vi "Main.vi"(11 "Module Admin":refnum<class "Delacor_lib_QMH_Module Admin.lvclass">) -> ()   [LabVIEW 2021, in "INSTR.lvlib"]
doc: "This template is based off of the Queued Message Handler design pattern and the Queued Message Handler project template that ships with LabVIEW.\n\nThe main difference is that the queue is private to this module and communication between modules is performed via Broadcast and Request events.\n\nRequest events are wrapped in public API methods and are handled in the Event Handling Loop (EHL) of this VI. Any module can register for Broadcast events sent by this module. The EHL generates messages based on user interface actions.\n\nThe Message Handling Loop (MHL) processes messages generated by the EHL, or by other messages. The messages are string values, so new messages can be added easily to the Message Cases case structure in the MHL. Each message cluster can also provide an optional value for Message Data, which is a variant that can be converted to whatever message-specific data is required.\n_____\nBased on Delacor QMH Project Template 5.0.0.82.\n\n<b>Note:</b> This VI was modified by the <b>Validate DQMH Module</b> tool to add a 'Panel Hidden' status updated broadcast to the Panel Close? event when External Launch = TRUE.\n\n<b>Note:</b> This VI was modified by the <b>Validate DQMH Module</b> tool to add a call to the Error Reported VI at the end of the 'Exit' MHL frame."
uses:
  INSTR.lvlib
  <vilib>/Delacor/Delacor QMH/Libraries/Module Admin_class/Delacor_lib_QMH_Module Admin.lvclass
  Module Data--cluster.ctl
  <vilib>/Delacor/Delacor QMH/Libraries/Message Queue_class/Delacor_lib_QMH_Message Queue.lvclass/Delacor_lib_QMH_Message Queue.ctl
  Stop Argument--cluster.ctl
  <vilib>/Delacor/Delacor QMH/Libraries/Module Admin_class/Delacor_lib_QMH_Module Admin.lvclass/Delacor_lib_QMH_Module Admin.ctl
  Simulation Argument--cluster.ctl
  <vilib>/Utility/miscctls.llb/LVPointTypeDef.ctl
  <vilib>/Delacor/Delacor QMH/Libraries/Message Queue_class/Delacor_lib_QMH_Enqueue Message (Single).vi
  <vilib>/Delacor/Delacor QMH/Libraries/Module Admin_class/Delacor_lib_QMH_Get External Launch.vi
  <vilib>/Utility/error.llb/Error Cluster From Error Code.vi
  <vilib>/ErrorRing/Error Ring.xnode
  <vilib>/Delacor/Delacor QMH/Libraries/Message Queue_class/Delacor_lib_QMH_Message Queue.lvclass
  <vilib>/DQMH Consortium/Lumos API/Libraries/SDV API/SDV API.lvlib
panel:
  out "ModuleName":string
  out "Sim?":bool
  in  "ExitMod":bool
  in  "Simulate MHL Error":bool
  in  "Simulate EHL Error":bool
  out "error out":errorcluster
  out "Status":string
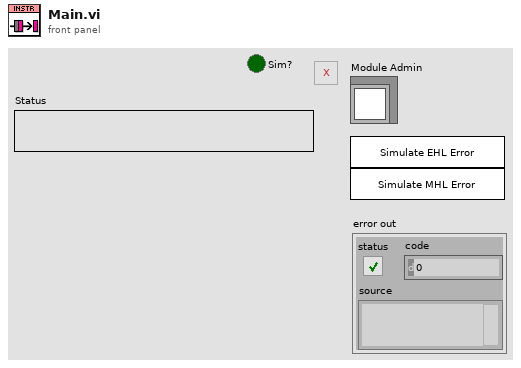
[diagram p1: front panel]
types:
  T1 = typedef "INSTR.lvlib/Request Events--cluster.ctl" = cluster{"Stop Module":refnum<user-event>, "Show Panel":refnum<user-event>, "Hide Panel":refnum<user-event>, "Get Module Execution Status":refnum<user-event>, "Show Diagram":refnum<user-event>, "Simulation":refnum<user-event>}
  T2 = typedef "INSTR.lvlib/Module Data--cluster.ctl" = cluster{"Status":string, "Sim":bool}
  T3 = enum32{"invalid lock state", "Not Locked", "Locked (No Password)", "Password-protected"}
  T4 = typedef "INSTR.lvlib/Stop Argument--cluster.ctl" = cluster{"Origin":string, "Exit via Stop Module Req?":bool, "Wait for Module to stop?":bool}
  T5 = typedef "INSTR.lvlib/Simulation Argument--cluster.ctl" = cluster{"Sim?":bool}
  T6 = typedef "LVPointTypeDef.ctl" = cluster{"Horizontal":i16, "Vertical":i16}
  T7 = enum32{"Invalid", "Standard", "Closed", "Hidden", "Minimized", "Maximized"}
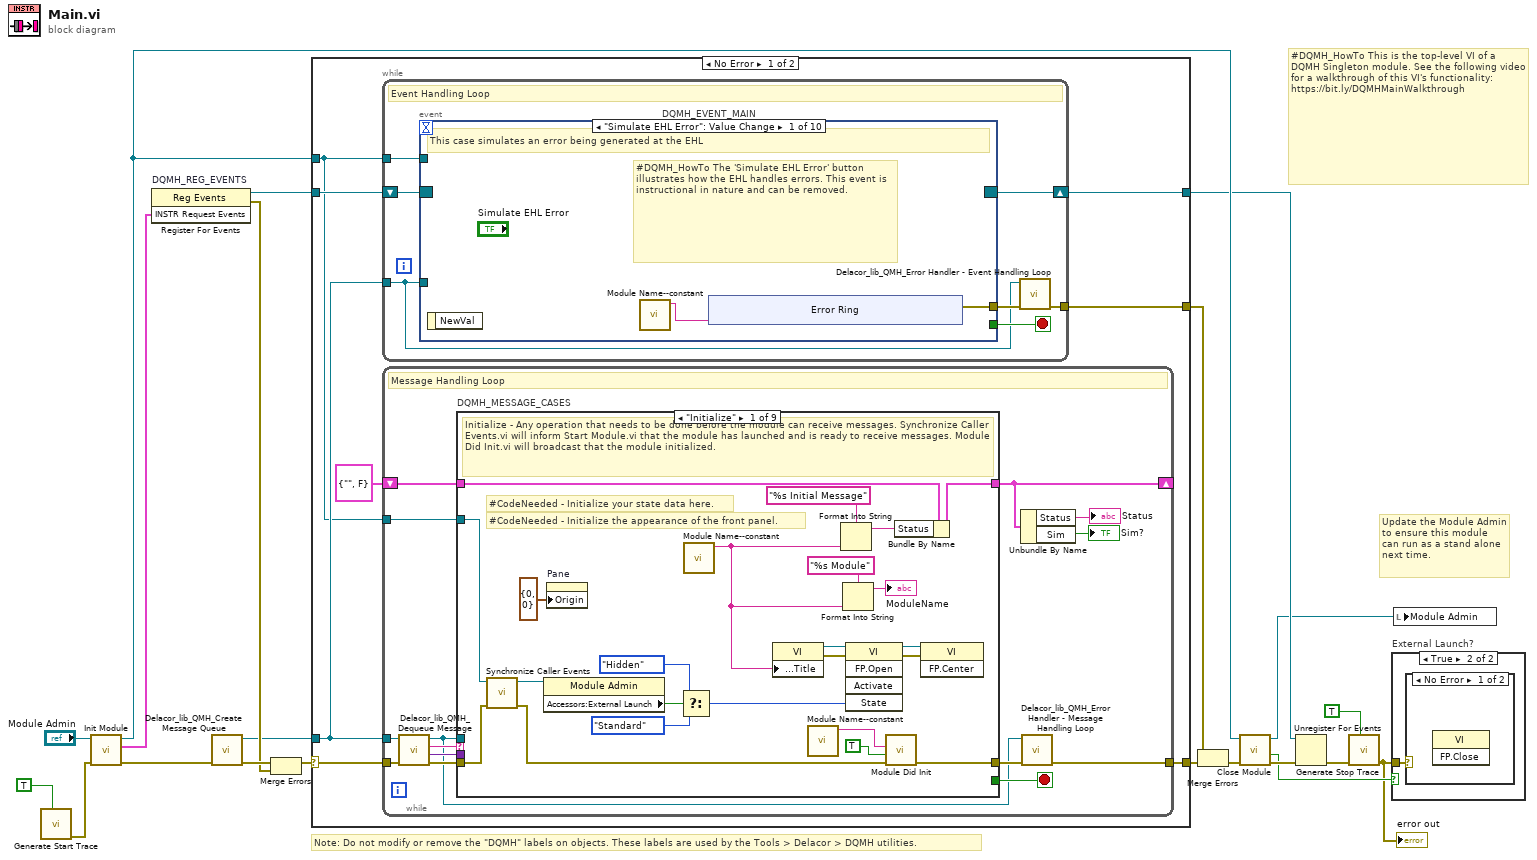
[diagram p0: block diagram]
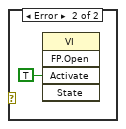
[diagram p3: hidden frame]
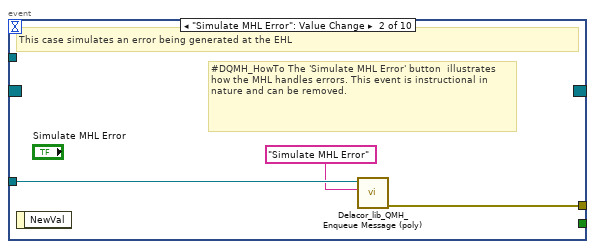
[diagram p4: hidden frame]
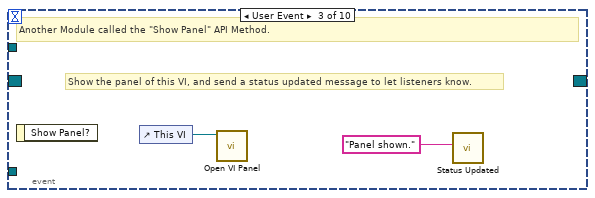
[diagram p5: hidden frame]
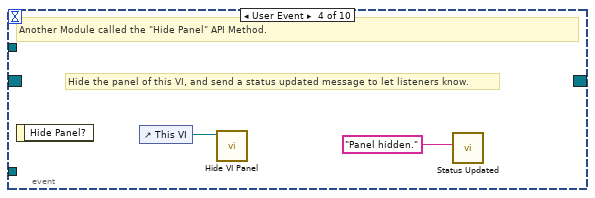
[diagram p6: hidden frame]
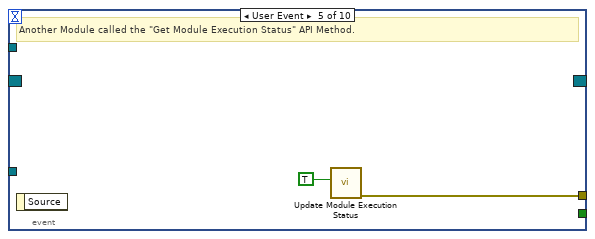
[diagram p7: hidden frame]
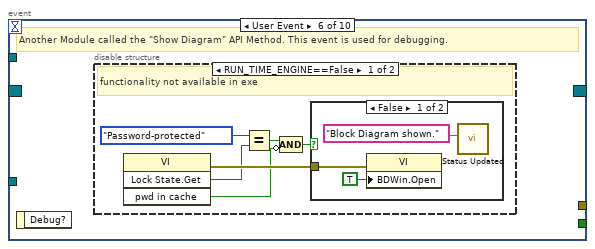
[diagram p8: hidden frame]
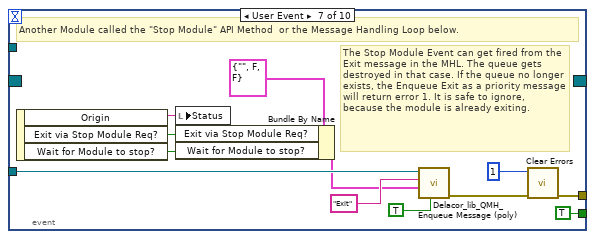
[diagram p11: hidden frame]
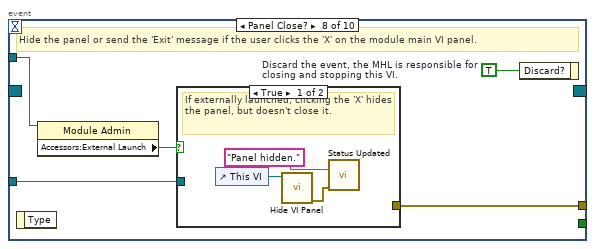
[diagram p12: hidden frame]
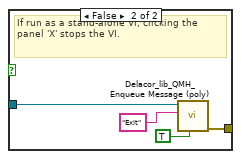
[diagram p13: hidden frame]
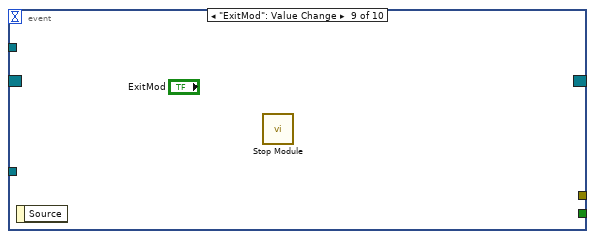
[diagram p14: hidden frame]
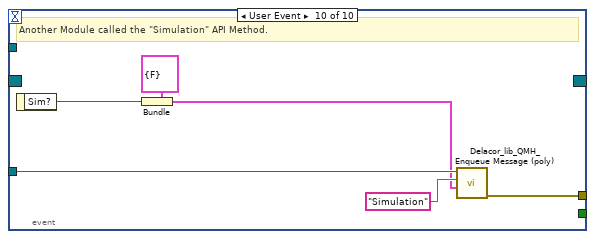
[diagram p15: hidden frame]
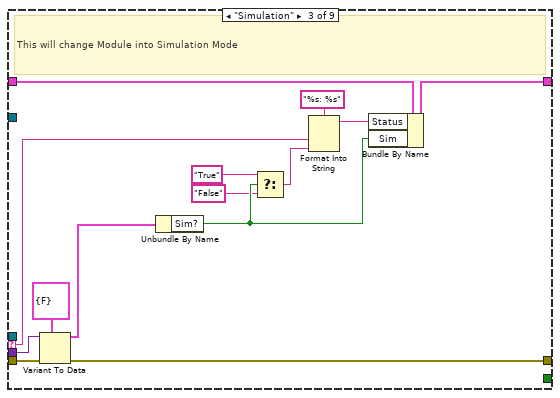
[diagram p17: hidden frame]
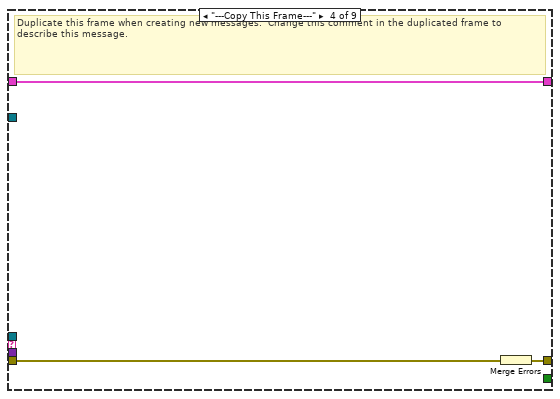
[diagram p18: hidden frame]
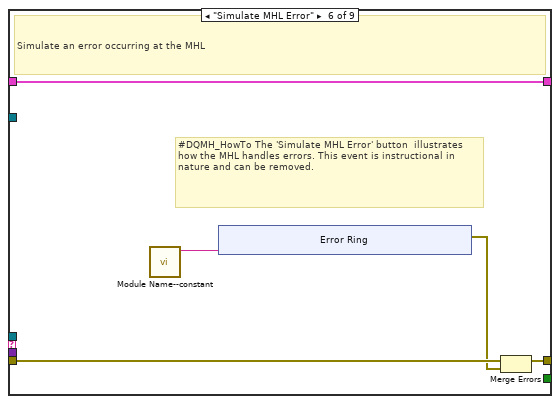
[diagram p20: hidden frame]
diagram:
  # "#DQMH_HowTo This is the top-level VI of a DQMH Singleton module. See the following video for a walkthrough of this VI's functionality: https://bit.ly/DQMHMainWalkthrough"
  # "Note: Do not modify or remove the \"DQMH\" labels on objects. These labels are used by the Tools > Delacor > DQMH utilities."
  # "Update the Module Admin to ensure this module can run as a stand alone next time."
  n1 = call <vilib>:"Generate Start Trace.vi"("Reply (F)"=TRUE) -> ("error out"=w4:errorcluster)  [unwired: 10 in]
  n2 = call "Init Module.vi"("error in (no error)"=w4, "Singleton Module Admin in"="Module Admin") -> ("error out"=w20:errorcluster, "INSTR Request Events"=w9:T1, "Singleton Module Admin out"=w12:refnum<class "Delacor_lib_QMH_Module Admin.lvclass">)  [unwired: 7 in]
  n3 = register-events "DQMH_REG_EVENTS"(w9) -> (reference out=w10:refnum<event-registration>, error out=w13:errorcluster)  [unwired: 2 in]
  n4 = call <vilib>:"Delacor_lib_QMH_Create Message Queue.vi"("error in"=w20) -> ("error out"=w15:errorcluster, "Message Queue"=w8:refnum<class "Delacor_lib_QMH_Message Queue.lvclass">)  [unwired: 9 in]
  n5 = Merge Errors(w15, w13) -> (w14:errorcluster)
  n6 = case shown="No Error" w14 {
    selector: w14 -> [w27 w211]
    tunnel: [w29 w210] -> w21
    tunnel: [w26 w216] -> w11
    tunnel: w10 -> [w24 w216]
    tunnel: w8 -> [w23 w209]
    tunnel: [w28 _] -> w18
    tunnel: w12 -> [w22 w212]
    frame No Error {
      n7 = while {
        tunnel: w23 -> [w30]
        shift-right: [w33] -> w26
        shift-left: w24 -> [w34]
        tunnel: [w35] -> w28
        tunnel: w22 -> [w31]
        stop <- w32 stop-if-true
        # "Event Handling Loop"
        n8 = event "DQMH_EVENT_MAIN" shown="[0] \"Simulate EHL Error\": Value Change" {
          selector: w34 -> [_ _ _ _ _ _ _ _ _ _]
          dyn-events: [_ _ _ _ _ _ _ _ _ _] -> w33
          timeout: _ -> [_ _ _ _ _ _ _ _ _ _]
          tunnel: [_ _ _ _ _ _ TRUE ("Discard?") _ _ _] -> w32
          tunnel: w30 -> [_ w47 _ _ _ _ w71 w78 _ w93]
          tunnel: [w38 w48 _ _ w54 _ w74 w80 _ w88] -> w36
          tunnel: w31 -> [_ _ _ _ _ _ _ w77 _ _]
          event "Simulate EHL Error": Value Change {
            # "#DQMH_HowTo The 'Simulate EHL Error' button  illustrates how the EHL handles errors. This event is instructional in nature and can be removed."
            # "This case simulates an error being generated at the EHL"
            n9 = event-data() -> ()  [unwired: 1 in, 1 out]
            n10 = call "Module Name--constant.vi"() -> ("Module Name"=w37:string)  [unwired: 11 in]
            n11 = xnode ("Error Ring")("parameter 0"=w37) -> ("error out"=w38:errorcluster)
          }
          event "Simulate MHL Error": Value Change {
            # "#DQMH_HowTo The 'Simulate MHL Error' button  illustrates how the MHL handles errors. This event is instructional in nature and can be removed."
            # "This case simulates an error being generated at the EHL"
            n12 = event-data() -> ()  [unwired: 1 in, 1 out]
            n13 = call-poly <vilib>:"Delacor_lib_QMH_Enqueue Message (poly).vi"("Message"="Simulate MHL Error", "Message Queue in"=w47) -> ("error out"=w48:errorcluster)  [unwired: 8 in, 1 out]
          }
          event User Event {
            # "Show the panel of this VI, and send a status updated message to let listeners know."
            # "Another Module called the \"Show Panel\" API Method."
            n14 = event-data() -> ()  [unwired: 1 in, 1 out]
            n15 = control-ref of="This VI"() -> (w50:refnum<vi>)
            n16 = call "Open VI Panel.vi"("VI"=w50) -> ()  [unwired: 10 in, 1 out]
            n17 = call "Status Updated.vi"("Status"="Panel shown." ("format string")) -> ()  [unwired: 10 in, 1 out]
          }
          event User Event {
            # "Hide the panel of this VI, and send a status updated message to let listeners know."
            # "Another Module called the \"Hide Panel\" API Method."
            n18 = event-data() -> ()  [unwired: 1 in, 1 out]
            n19 = control-ref of="This VI"() -> (w52:refnum<vi>)
            n20 = call "Hide VI Panel.vi"("VI"=w52) -> ()  [unwired: 10 in, 1 out]
            n21 = call "Status Updated.vi"("Status"="Panel hidden." ("format string")) -> ()  [unwired: 10 in, 1 out]
          }
          event User Event {
            # "Another Module called the \"Get Module Execution Status\" API Method."
            n22 = event-data() -> ()  [unwired: 1 in, 1 out]
            n23 = call "Update Module Execution Status.vi"("Running?"=TRUE) -> ("error out"=w54:errorcluster)  [unwired: 10 in]
          }
          event User Event {
            # "Another Module called the \"Show Diagram\" API Method. This event is used for debugging."
            n24 = event-data() -> ()  [unwired: 1 in, 1 out]
            n25 = disable-structure "Conditional Disable Structure" shown="RUN_TIME_ENGINE==False" {
              frame condition #0 (active) {
                # "functionality not available in exe"
                n26 = invoke on="Invoke Node" class="VI" method="Lock State.Get"() -> (error out=w60:errorcluster, "Get Lock State"=w59:T3, "pwd in cache"=w56:bool)  [unwired: 4 in, 1 out]
                n27 = Equal?(x=T3."Password-protected", y=w59) -> (x = y?=w57:bool)
                n28 = Compound Arithmetic op=AND(w57, invert w56) -> (w55:bool)
                n29 = case shown="False" w55 {
                  tunnel: w60 -> [w63 _]
                  frame False {
                    n30 = property on="Property Node" class="VI"(error in=w63, "BDWin.Open"=TRUE ("Block Diagram Window:Open")) -> ()  [unwired: 1 in, 2 out]
                    n31 = call "Status Updated.vi"("Status"="Block Diagram shown." ("format string")) -> ()  [unwired: 10 in, 1 out]
                  }
                  frame True {
                    # "Password-protected VI, and the password is not in the cache. Do not show the diagram."
                  }
                }
              }
              frame condition #1 {
              }
            }
          }
          event User Event {
            # "The Stop Module Event can get fired from the Exit message in the MHL. The queue gets destroyed in that case. If the queue no longer exists, the Enqueue Exit as a priority message will return error 1. It is safe to ignore, because the module is already exiting."
            # "Another Module called the \"Stop Module\" API Method  or the Message Handling Loop below."
            n32 = event-data() -> ("Origin"=w70:string, "Exit via Stop Module Req?"=w66:bool, "Wait for Module to stop?"=w65:bool)  [unwired: 1 in]
            n33 = local write "Status"(w70) -> ()
            n34 = Bundle By Name(cluster=T4 {"Origin"="", "Exit via Stop Module Req?"=FALSE, "Wait for Module to stop?"=FALSE} ("Stop Argument"), "Exit via Stop Module Req?"=w66, "Wait for Module to stop?"=w65) -> (w64:T4)
            n35 = call-poly <vilib>:"Delacor_lib_QMH_Enqueue Message (poly).vi"("Priority Message? (F)"=TRUE, "Message Data"=w64, "Message"="Exit", "Message Queue in"=w71) -> ("error out"=w75:errorcluster)  [unwired: 6 in, 1 out]
            n36 = call <vilib>:"Clear Errors.vi"("error in (no error)"=w75, "specific error code to clear (0: all)"=1) -> ("error out"=w74:errorcluster)  [unwired: 4 in, 1 out]
          }
          event Panel Close? {
            w79 = TRUE  # Discard the event, the MHL is responsible for closing and stopping this VI.
            # "Hide the panel or send the 'Exit' message if the user clicks the 'X' on the module main VI panel."
            n37 = event-data() -> ()  [unwired: 1 in, 1 out]
            n38 = property on="Property Node" class="Module Admin"(reference=w77) -> ("Accessors:External Launch"=w76:bool)  [unwired: 1 in, 2 out]
            n39 = case shown="True" w76 {
              tunnel: w78 -> [_ w86]
              tunnel: [_ w87] -> w80
              frame True {
                # "If externally launched, clicking the 'X' hides the panel, but doesn't close it."
                n40 = control-ref of="This VI"() -> (w83:refnum<vi>)
                n41 = call "Hide VI Panel.vi"("VI"=w83) -> ("error out"=w81:errorcluster)  [unwired: 10 in]
                n42 = call "Status Updated.vi"("error in (no error)"=w81, "Status"="Panel hidden.") -> ()  [unwired: 9 in, 1 out]
              }
              frame False {
                # "If run as a stand-alone VI, clicking the panel 'X' stops the VI."
                n43 = call-poly <vilib>:"Delacor_lib_QMH_Enqueue Message (poly).vi"("Priority Message? (F)"=TRUE, "Message"="Exit", "Message Queue in"=w86) -> ("error out"=w87:errorcluster)  [unwired: 7 in, 1 out]
              }
            }
            n44 = event-data ("Event Filter Node")("Discard?"=w79) -> ()  [unwired: 1 in, 1 out]
          }
          event "ExitMod": Value Change {
            n45 = event-data() -> ()  [unwired: 1 in, 1 out]
            n46 = call "Stop Module.vi"() -> ()  [unwired: 11 in, 1 out]
          }
          event User Event {
            # "Another Module called the \"Simulation\" API Method."
            n47 = event-data() -> ("Sim?"=w89:bool)  [unwired: 1 in]
            n48 = Bundle(cluster=T5 {"Sim?"=FALSE} ("Simulation Argument"), "Sim?"=w89) -> (w90:T5)
            n49 = call-poly <vilib>:"Delacor_lib_QMH_Enqueue Message (poly).vi"("Message Data"=w90, "Message"="Simulation", "Message Queue in"=w93) -> ("error out"=w88:errorcluster)  [unwired: 7 in, 1 out]
          }
        }
        n50 = call-dynamic "Delacor_lib_QMH_Error Handler - Event Handling Loop.vi"("error in"=w36, "Message Queue in"=w30) -> ("dup error in"=w35:errorcluster)  [unwired: 8 in, 1 out]
      }
      n51 = while {
        tunnel: w23 -> [w99]
        shift-right: [w96] -> _
        shift-left: T2 {"Status"="", "Sim"=FALSE} ("Data Cluster") -> [w103]
        tunnel: w27 -> [w106]
        tunnel: [w104] -> w29
        tunnel: w22 -> [w97]
        stop <- w102 stop-if-true
        # "Message Handling Loop"
        n52 = call-dynamic "Delacor_lib_QMH_Dequeue Message.vi"("error in"=w106, "Message Queue in"=w99) -> ("error out"=w105:errorcluster, "Message Data"=w100:variant, "Message"=w101:string, "Message Queue out"=w98:refnum<class "Delacor_lib_QMH_Message Queue.lvclass">)  [unwired: 6 in]
        n53 = case "DQMH_MESSAGE_CASES" shown="\"Initialize\"" w101 {
          selector: w101 -> [_ _ w139 _ _ _ _ _ w196]
          tunnel: w98 -> [_ _ _ _ _ _ w166 w188 _]
          tunnel: w105 -> [w128 w132 w146 w149 w151 w156 w173 w194 w198]
          tunnel: [w126 w132 w144 w148 w151 w155 w169 w191 w199] -> w107
          tunnel: w103 -> [w118 w131 w145 w147 w150 w153 w168 w187 w197]
          tunnel: [w117 w131 w140 w147 w150 w153 w168 w187 w197] -> w96
          tunnel: [_ _ _ _ _ _ _ w186 _] -> w102
          tunnel: w100 -> [_ _ w143 _ _ _ w167 w185 _]
          tunnel: w97 -> [w119 _ _ _ _ _ w165 w180 _]
          frame "Initialize" {
            # "#CodeNeeded - Initialize the appearance of the front panel."
            # "#CodeNeeded - Initialize your state data here."
            # "Initialize - Any operation that needs to be done before the module can receive messages. Synchronize Caller Events.vi will inform Start Module.vi that the module has launched and is ready to receive messages. Module Did Init.vi will broadcast that the module initialized."
            n54 = call "Synchronize Caller Events.vi"("error in (no error)"=w128, "Singleton Module Admin in"=w119) -> ("error out"=w127:errorcluster, "Singleton Module Admin out"=w114:refnum<class "Delacor_lib_QMH_Module Admin.lvclass">)  [unwired: 8 in]
            n55 = property on="Property Node" class="Module Admin"(reference=w114) -> ("Accessors:External Launch"=w123:bool)  [unwired: 1 in, 2 out]
            n56 = property on="Pane" class="Pane"("Origin"=T6 {"Horizontal"=0, "Vertical"=0}) -> ()  [unwired: 2 in, 2 out]
            n57 = Select(t=T7."Hidden" ("State"), s=w123, f=T7."Standard" ("State")) -> (s? t:f=w120:T7)
            n58 = call "Module Name--constant.vi"() -> ("Module Name"=w110:string)  [unwired: 11 in]
            n59 = property on="Property Node" class="VI"("Front Panel.Title"=w110) -> (reference out=w125:refnum<vi>, error out=w130:errorcluster)  [unwired: 2 in]
            n60 = call "Module Name--constant.vi"() -> ("Module Name"=w115:string)  [unwired: 11 in]
            n61 = Format Into String(format string="%s Initial Message" ("Initial Message"), w110) -> (resulting string=w112:string)  [unwired: 2 in, 1 out]
            n62 = Format Into String(format string="%s Module", w110) -> (resulting string=→"ModuleName":string)  [unwired: 2 in, 1 out]
            n63 = invoke on="Invoke Node" class="VI" method="FP.Open"(reference=w125, error in=w130, "State"=w120) -> (reference out=w124:refnum<vi>, error out=w129:errorcluster)  [unwired: 2 in, 3 out]
            n64 = call "Module Did Init.vi"("error in (no error)"=w127, "Initialized?"=TRUE, "Origin"=w115) -> ("error out"=w126:errorcluster)  [unwired: 8 in]
            n65 = Bundle By Name(cluster=w118, "Status"=w112) -> (w117:T2)
            n66 = invoke on="Invoke Node" class="VI" method="FP.Center"(reference=w124, error in=w129) -> ()  [unwired: 1 in, 3 out]
          }
          frame "--- Module Specific ---" {
            # "Separator -- The following cases handle messages specific to this Module."
          }
          frame "Simulation" {
            # "This will change Module into Simulation Mode"
            n67 = Variant To Data(error in=w146, type=T5 {"Sim?"=FALSE} ("Simulation Argument"), Variant=w143) -> (data=w141:T5, error out=w144:errorcluster)
            n68 = Unbundle By Name(w141) -> ("Sim?"=w138:bool)
            n69 = Select(t="True", s=w138, f="False") -> (s? t:f=w134:string)
            n70 = Format Into String(format string="%s: %s", w139, w134) -> (resulting string=w133:string)  [unwired: 2 in, 1 out]
            n71 = Bundle By Name(cluster=w145, "Status"=w133, "Sim"=w138) -> (w140:T2)
          }
          frame "---Copy This Frame---" {
            # "Duplicate this frame when creating new messages.  Change this comment in the duplicated frame to describe this message."
            n72 = Merge Errors(w149) -> (w148:errorcluster)
          }
          frame "--- Exit and Error Handling---" {
            # "Separator - The following cases handle errors and exit messages."
          }
          frame "Simulate MHL Error" {
            # "#DQMH_HowTo The 'Simulate MHL Error' button  illustrates how the MHL handles errors. This event is instructional in nature and can be removed."
            # "Simulate an error occurring at the MHL"
            n73 = call "Module Name--constant.vi"() -> ("Module Name"=w152:string)  [unwired: 11 in]
            n74 = xnode ("Error Ring")("parameter 0"=w152) -> ("error out"=w154:errorcluster)
            n75 = Merge Errors(w156, w154) -> (w155:errorcluster)
          }
          frame "Error" {
            # "#CodeRecommended - If you ever change the name of this \"Error\" message, you'll need to update the name in the Check Loop Error.vi as well."
            # "#CodeRecommended - If the module is running in standalone mode (External Launch = FALSE), this code will pop up an error dialog and call the 'Exit' message if an error occurs. Add more fine-grained error handling here."
            # "Error - Check the error message data and respond accordingly. This message is sent by the \"Error Handler\" VIs at the end of each loop in this application."
            n76 = property on="Property Node" class="Module Admin"(reference=w165) -> ("Accessors:External Launch"=w164:bool)  [unwired: 1 in, 2 out]
            n77 = Variant To Data(error in=w173, type=errorcluster {"status"=FALSE, "code"=0, "source"=""} ("error constant"), Variant=w167) -> (data=w174:errorcluster, error out=w171:errorcluster)
            n78 = call "Error Reported.vi"("Error"=w174) -> ()  [unwired: 10 in, 1 out]
            n79 = case shown="False" w164 {
              tunnel: [w179 _] -> w170
              tunnel: w166 -> [w177 _]
              tunnel: w174 -> [w178 _]
              frame False {
                # "If the module is running standalone, then pop up an error dialog and call the \"Exit\" message."
                n80 = call <vilib>:"Simple Error Handler.vi"("error in (no error)"=w178) -> ()  [unwired: 4 in, 5 out]
                n81 = call-poly <vilib>:"Delacor_lib_QMH_Enqueue Message (poly).vi"("Priority Message? (F)"=TRUE, "Message"="Exit", "Message Queue in"=w177) -> ("error out"=w179:errorcluster)  [unwired: 7 in, 1 out]
              }
              frame True {
                # "If the module was launched externally, calling the Error Reported broadcast VI is the only action performed by the \"Error\" message. The module's caller can then process the error appropriately."
              }
            }
            n82 = Merge Errors(w171, w170) -> (w169:errorcluster)
            n83 = local write "error out"(w169) -> ()
          }
          frame "Exit" {
            w184 = 91  # 91: not all Exit messages will have an argument
            w186 = TRUE  # Stop the VI
            # "Release the message queue reference"
            # "#CodeNeeded - Add any required cleanup code here"
            # "Exit - Exit the application."
            n84 = Variant To Data(error in=w194, type=T4 {"Origin"="", "Exit via Stop Module Req?"=FALSE, "Wait for Module to stop?"=FALSE} ("Stop Argument"), Variant=w185) -> (data=w182:T4, error out=w190:errorcluster)
            n85 = call <vilib>:"Clear Errors.vi"("error in (no error)"=w190, "specific error code to clear (0: all)"=w184) -> ("error out"=w193:errorcluster)  [unwired: 4 in, 1 out]
            n86 = control-ref of="This VI"() -> (w181:refnum<vi>)
            n87 = call-dynamic "Delacor_lib_QMH_Release Message Queue.vi"("error in"=w193, "Message Queue"=w188) -> ("error out"=w192:errorcluster)  [unwired: 9 in]
            n88 = call "Handle Exit.vi"("Stop Argument"=w182, "Admin in"=w180, "VI reference"=w181) -> ("error out"=w189:errorcluster)  [unwired: 7 in, 1 out]
            n89 = Merge Errors(w192, w189) -> (w191:errorcluster)
            n90 = call "Error Reported.vi"("Error"=w191) -> ()  [unwired: 10 in, 1 out]
          }
          frame Default {
            # "'Default' case only runs if there is a message that isn't defined in any of the other cases.  Output a programming error."
            n91 = call "Module Name--constant.vi"() -> ("Module Name"=w195:string)  [unwired: 11 in]
            n92 = xnode ("Error Ring")("parameter 0"=w196, "parameter 1"=w195) -> ("error out"=w200:errorcluster)
            n93 = Merge Errors(w198, w200) -> (w199:errorcluster)
          }
        }
        n94 = Unbundle By Name(w96) -> ("Status"=→"Status":string, "Sim"=→"Sim?":bool)
        n95 = call-dynamic "Delacor_lib_QMH_Error Handler - Message Handling Loop.vi"("error in"=w107, "Message Queue in"=w98) -> ("dup error in"=w104:errorcluster)  [unwired: 8 in, 1 out]
      }
    }
    frame Error {
      # "Synchronize Caller Events.vi will inform Start Module.vi that the module has launched and will let the code calling Start Module.vi register for broadcasts and would permit the caller receive the broadcast that an error occurred at launch time."
      n96 = call-dynamic "Delacor_lib_QMH_Release Message Queue.vi"("error in"=w211, "Message Queue"=w209) -> ("error out"=w210:errorcluster)  [unwired: 9 in]
      n97 = call "Synchronize Caller Events.vi"("Singleton Module Admin in"=w212) -> ("error out"=w217:errorcluster)  [unwired: 9 in, 1 out]
      n98 = call "Module Name--constant.vi"() -> ("Module Name"=w215:string)  [unwired: 11 in]
      n99 = Format Into String(format string="An error occurred during initialization. %s is no longer running.", w215) -> (resulting string=w213:string)  [unwired: 2 in, 1 out]
      n100 = Merge Errors(w210, w217) -> (w218:errorcluster)
      n101 = call "Error Reported.vi"("Additional Information"=w213, "Error"=w218) -> ()  [unwired: 9 in, 1 out]
    }
  }
  n102 = Merge Errors(w18, w21) -> (w17:errorcluster)
  n103 = call "Close Module.vi"("error in (no error)"=w17, "Module Admin in"=w12) -> ("error out"=w19:errorcluster, "External Launch"=w5:bool, "Module Admin out"=w6:refnum<class "Delacor_lib_QMH_Module Admin.lvclass">)  [unwired: 7 in]
  n104 = Unregister For Events(event registration refnum=w11, error in=w19) -> (error out=w16:errorcluster)
  n105 = call <vilib>:"Generate Stop Trace.vi"("Reply (F)"=TRUE, "error in (no error)"=w16) -> ("error out"=w2:errorcluster)  [unwired: 9 in]
  "error out" <- w2
  n106 = case "External Launch?" shown="True" w5 {
    tunnel: w2 -> [_ w219]
    frame False {
    }
    frame True {
      n107 = case shown="No Error" w219 {
        frame No Error {
          n108 = invoke on="Invoke Node" class="VI" method="FP.Close"() -> ()  [unwired: 3 in, 3 out]
        }
        frame Error {
          n109 = invoke on="Invoke Node" class="VI" method="FP.Open"("Activate"=TRUE ("Activate?")) -> ()  [unwired: 4 in, 5 out]
        }
      }
    }
  }
  n110 = local write "Module Admin"(w6) -> ()
